vi "Initialize SLSC Switch Custom Device.vi"(8 "error in (no error)":errorcluster, 11 "SLSC Switch Custom Device Ref in":T1 format="%.0x") -> (0 "error out":errorcluster, 2 "Endpoint Configuration Section Ref":T1 format="%.0x", 3 "SLSC Switch Custom Device Ref out":T1 format="%.0x")   [LabVIEW 2017, in "SLSC Switch Scripting.lvlib"]
uses:
  SLSC Switch Scripting.lvlib
  <vilib>/NI Veristand/Custom Device API/Custom Device Item Ref.ctl
  Properties/SLSC Switch All Properties.ctl
  SLSC Scripting Constants.vi
  Shared/Constants.vi
  <vilib>/NI Veristand/Custom Device API/Custom Device API.lvlib
  Shared/SLSC Switch Shared.lvlib
  Shared/Routing and Faulting Consumer System Definition API/Routing and Faulting Hardware API.lvlib
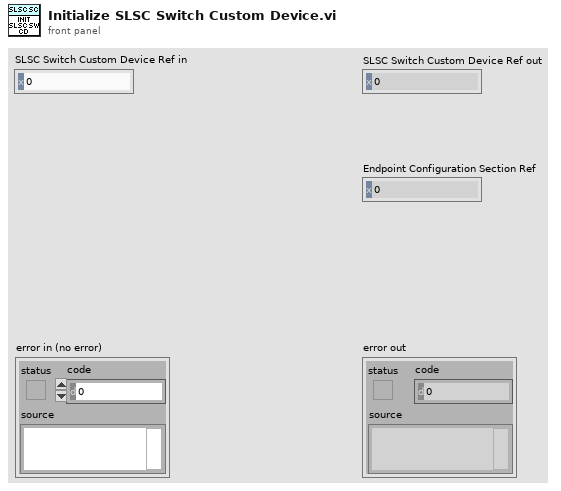
[diagram p1: front panel]
types:
  T1 = typedef "Custom Device API.lvlib/Custom Device Item Ref.ctl" = u64
  T2 = typedef "SLSC Switch Scripting.lvlib/SLSC Switch All Properties.ctl" = cluster{"Model":string, "Resource":string, "Topology":string, "Capabilities":string, "Description":string}
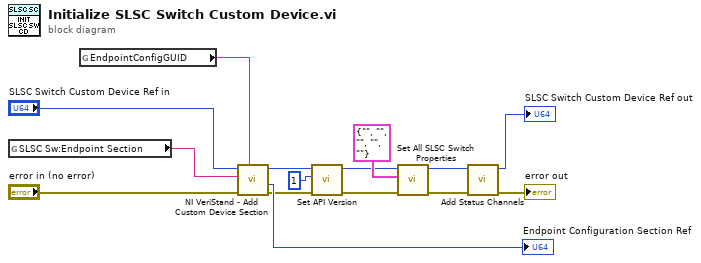
[diagram p0: block diagram]
diagram:
  n1 = global read "SLSC Scripting Constants.vi" "SLSC Sw:Endpoint Section"() -> (w13:string)
  n2 = global read "Constants.vi" "EndpointConfigGUID"() -> (w10:string)
  n3 = call <vilib>:"NI VeriStand - Add Custom Device Section.vi"("GUID (Default Section)"=w10, "error in (no error)"="error in (no error)", "Section Name"=w13, "Parent Ref in"="SLSC Switch Custom Device Ref in") -> ("error out"=w4:errorcluster, "Section Ptr"=→"Endpoint Configuration Section Ref":T1, "Parent Ref out"=w5:T1)  [unwired: 4 in, 1 out]
  n4 = call "Set API Version.vi"("error in (no error)"=w4, "API version"=1, "Hardware Ref in"=w5) -> ("error out"=w3:errorcluster, "Hardware Ref out"=w2:T1)  [unwired: 7 in]
  n5 = call "Set All SLSC Switch Properties.vi"("error in (no error)"=w3, "SLSC Switch All Properties"=T2 {"Model"="", "Resource"="", "Topology"="", "Capabilities"="", "Description"=""}, "SLSC Switch Custom Device Ref in"=w2) -> ("error out"=w9:errorcluster, "SLSC Switch Custom Device Ref out"=w7:T1)  [unwired: 7 in]
  n6 = call "Add Status Channels.vi"("error in (no error)"=w9, "SLSC Switch Custom Device Ref in"=w7) -> ("error out"=→"error out":errorcluster, "SLSC Switch Custom Device Ref out"=→"SLSC Switch Custom Device Ref out":T1)  [unwired: 8 in]
